vi "CHECK Color V3.vi"(8 "error in (no error)":errorcluster, 11 "refnum name":string) -> (0 "error out":errorcluster, 1 "Proximity":u16, 2 "Matched Color Name":string, 3 "ColorSensorDevRef out":T1={"I2CDevRef"={"DevStatus"={"status"=FALSE, "code"=0, "source"=""}, "Device Address"=0, "Handle"=0, "I2C Bus"=enum."Invalid"}} {"I2CDevRef"."Device Address" format="%.0x"}, 4 "Confidence":dbl)   [LabVIEW 2020]
uses:
  <vilib>/Rock Robotics/WPI/ThirdParty/REV Robotics/REVLib/Typedef/Color Sensor V3 DevRef.ctl
  <vilib>/Rock Robotics/WPI/I2C/WPI_I2CDevRef.ctl
  <vilib>/Rock Robotics/SystemInterfaces/i2clib/i2c_bus.ctl
  <vilib>/Rock Robotics/Network Tables/NT Write String.vi
  <vilib>/Rock Robotics/Network Tables/NT Write Number.vi
  <vilib>/Rock Robotics/Network Tables/NT Write Numeric Array.vi
panel:
  out "Matched Color":cluster{"R":dbl, "G":dbl, "B":dbl}
  out "Normalized Color":cluster{"R":dbl, "G":dbl, "B":dbl}
  out "Color":u32(colorbox)
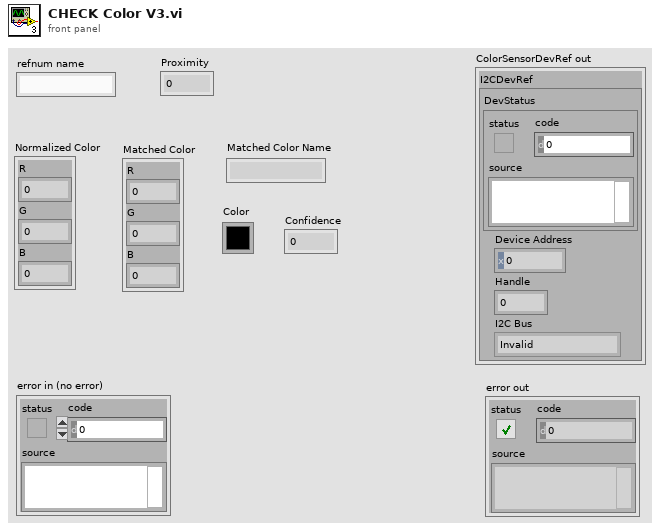
[diagram p1: front panel]
types:
  T1 = typedef "Color Sensor V3 DevRef.ctl" = cluster{"I2CDevRef":T2}
  T2 = typedef "WPI_I2CDevRef.ctl" = cluster{"DevStatus":errorcluster, "Device Address":u8, "Handle":i32, "I2C Bus":T3}
  T3 = typedef "i2c_bus.ctl" = enum16{"I2C On-Board", "I2C MXP", "Invalid"}
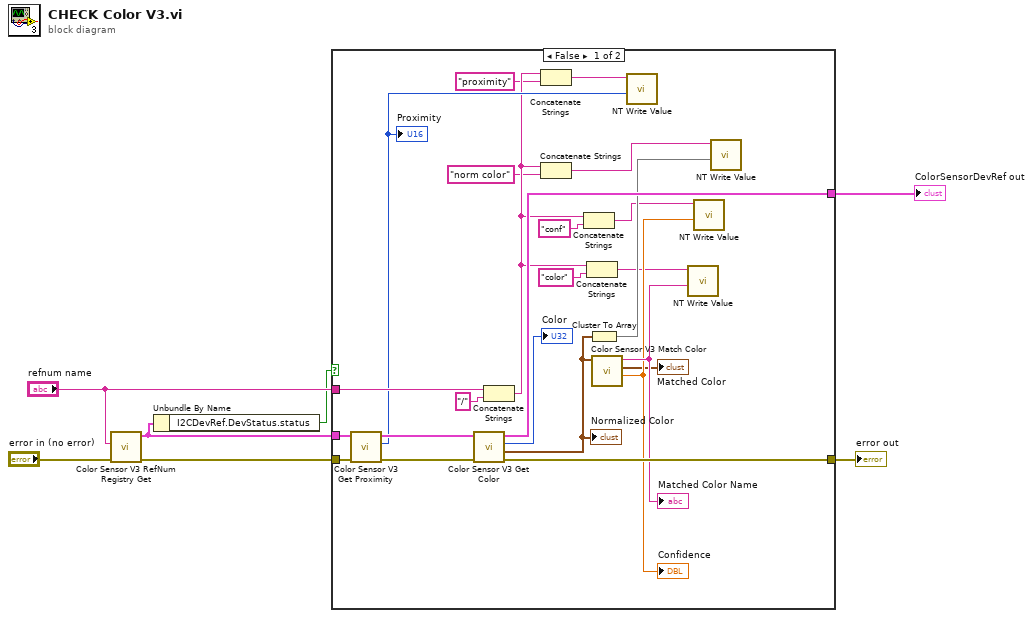
[diagram p0: block diagram]
diagram:
  n1 = call <vilib>:"Color Sensor V3 RefNum Registry Get.vi"("error in (no error)"="error in (no error)", "refnum name"="refnum name") -> ("error out"=w3:errorcluster, "ColorSensorDevRef"=w2:T1)  [unwired: 8 in]
  n2 = Unbundle By Name(w2) -> ("I2CDevRef.DevStatus.status"=w1:bool)
  n3 = case shown="False" w1 {
    tunnel: "refnum name" -> [w31 _]
    tunnel: [w30 _] -> w6
    tunnel: [w29 _] -> w5
    tunnel: w3 -> [w28 _]
    tunnel: w2 -> [w27 _]
    frame False {
      n4 = call <vilib>:"Color Sensor V3 Get Proximity.vi"("error in (no error)"=w28, "ColorSensorDevRef"=w27) -> ("error out"=w26:errorcluster, "Proximity"=w24:u16, "ColorSensorDevRef out"=w25:T1)  [unwired: 7 in]
      "Proximity" <- w24
      n5 = call <vilib>:"Color Sensor V3 Get Color.vi"("error in (no error)"=w26, "ColorSensorDevRef"=w25) -> ("error out"=w30:errorcluster, "Normalized Color"=w21:cluster{"R":dbl, "G":dbl, "B":dbl}, "Color"=→"Color":u32, "ColorSensorDevRef out"=w29:T1)  [unwired: 6 in]
      "Normalized Color" <- w21
      n6 = Concatenate Strings(w31, "/" ("string")) -> (w19:string)
      n7 = Concatenate Strings(w19, "proximity" ("string")) -> (w17:string)
      n8 = Concatenate Strings(w19, "norm color" ("string")) -> (w16:string)
      n9 = Concatenate Strings(w19, "conf" ("string")) -> (w15:string)
      n10 = Concatenate Strings(w19, "color" ("string")) -> (w14:string)
      n11 = Cluster To Array(cluster=w21) -> (array=w20:dbl[])
      n12 = call <vilib>:"Color Sensor V3 Match Color.vi"("Measured Color"=w21) -> ("Confidence"=w22:dbl, "Matched Color"=→"Matched Color":cluster{"R":dbl, "G":dbl, "B":dbl}, "Matched Color Name"=w23:string)  [unwired: 8 in]
      "Confidence" <- w22
      "Matched Color Name" <- w23
      n13 = call-poly <vilib>:"NT Write Value.vi"("Numeric"=w24, "Name"=w17) -> ()  [unwired: 9 in, 1 out]
      n14 = call-poly <vilib>:"NT Write Value.vi"("String"=w23, "Name"=w14) -> ()  [unwired: 9 in, 1 out]
      n15 = call-poly <vilib>:"NT Write Value.vi"("Numeric"=w22, "Name"=w15) -> ()  [unwired: 9 in, 1 out]
      n16 = call-poly <vilib>:"NT Write Value.vi"("Numeric Array"=w20, "Name"=w16) -> ()  [unwired: 9 in, 1 out]
    }
    frame True {
    }
  }
  "error out" <- w6
  "ColorSensorDevRef out" <- w5
